vi "SplineParam_StackPush.vi"(9 "T1":dbl, 10 "T0":dbl, 11 "InputStack":T1) -> (3 "OutputStack":T1)   [LabVIEW 2019, in "Trajectory_Library.lvlib"]
doc: "Internal routine used by SplineParam_Spline_T0_T1. This routine \"pushes\" the item to the top of the stack and increments the number of items on the stack.\n\nParameters:\n - InputStack - Stack data structure\n - T0\n - T1\nReturns:\n - OutputStack - Updated Stack data structure"
uses:
  Trajectory_Library.lvlib
  PARAM_STACK.ctl
  PARAM_STACK_ITEM.ctl
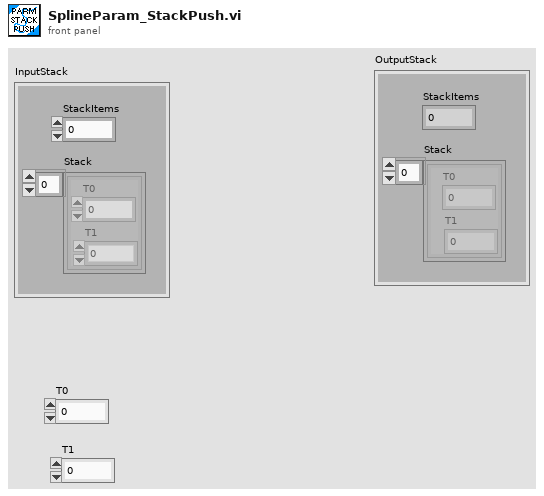
[diagram p1: front panel]
types:
  T1 = typedef "Trajectory_Library.lvlib/PARAM_STACK.ctl" = cluster{"StackItems":i32, "Stack":T2[]}
  T2 = typedef "Trajectory_Library.lvlib/PARAM_STACK_ITEM.ctl" = cluster{"T0":dbl, "T1":dbl}
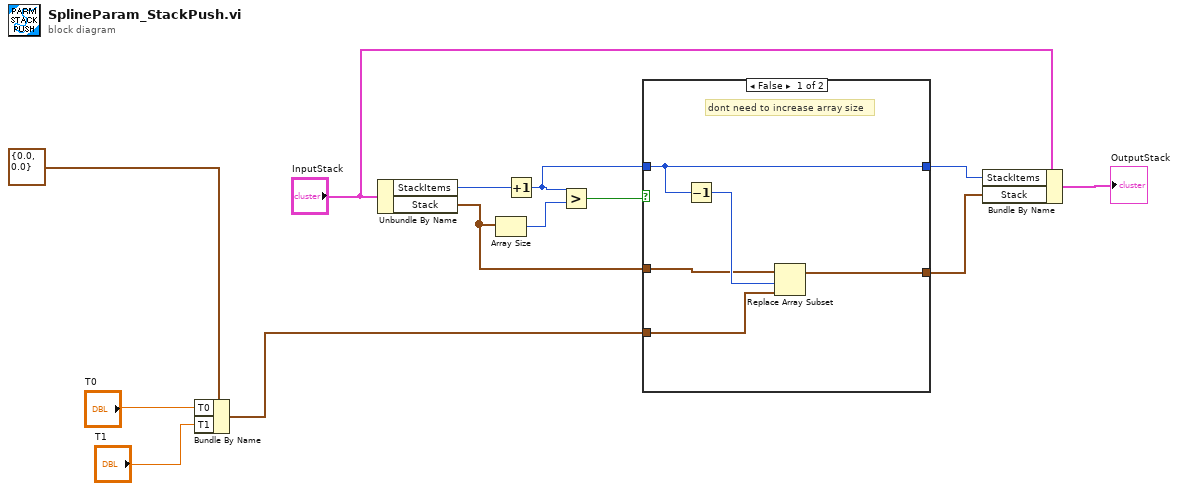
[diagram p0: block diagram]
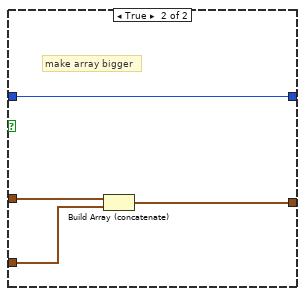
[diagram p2: hidden frame]
diagram:
  n1 = Bundle By Name(cluster=T2 {"T0"=0.0, "T1"=0.0} ("PARAM_STACK"), "T0"="T0", "T1"="T1") -> (w1:T2)
  n2 = Unbundle By Name("InputStack") -> ("StackItems"=w13:i32, "Stack"=w10:T2[])
  n3 = Array Size(array=w10) -> (size(s)=w12:i32)
  n4 = Increment(x=w13) -> (x+1=w9:i32)
  n5 = Greater?(x=w9, y=w12) -> (0:w11:bool)
  n6 = case shown="False" w11 {
    tunnel: w10 -> [w16 w22]
    tunnel: w1 -> [w15 w21]
    tunnel: [w14 w20] -> w7
    tunnel: w9 -> [w18 w19]
    tunnel: [w18 w19] -> w6
    frame False {
      # "dont need to increase array size"
      n7 = Decrement(x=w18) -> (x-1=w17:i32)
      n8 = Replace Array Subset(array=w16, new element=w15, index=w17) -> (w14:T2[])
    }
    frame True {
      # "make array bigger"
      n9 = Build Array (concatenate)(w22, w21) -> (w20:T2[])
    }
  }
  n10 = Bundle By Name(cluster="InputStack", "StackItems"=w6, "Stack"=w7) -> (→"OutputStack":T1)
